vi "Update Graphs.vi"(0 "Select Graph":T15, 2 "appended array":refnum<vi>[](array[refnum]), 5 "ERD Graph  Ind 2":T14, 7 "ERD_Data_Bundled_In":T1, 11 "Error In":errorcluster) -> (1 "All Loads":u16[][](graph), 3 "Water Temperature":dbl(graph), 4 "Basket Speed":u16[][](graph), 6 "Tub Gallons":dbl(graph), 8 "Pressure":dbl(graph), 10 "Motor Current":dbl(graph), 12 "ERD 3":dbl(graph), 13 "ERD 2":dbl(graph), 14 "ERD 1":dbl(graph), 15 "Error Out":errorcluster)   [LabVIEW 2021]
doc: "This VI displays (makes visable) the corresponding graph based on user selection, as well as updates the values of the graphs with current data."
uses:
  type defs/Select _Graph.ctl
  type defs/All_Bundled_Data.ctl
  type defs/Version.ctl
  type defs/ERD_Always_Show.ctl
  type defs/Brass Matrix.ctl
  type defs/CSV_File_String_Arrays.ctl
  type defs/Redundant.ctl
  type defs/Algorithms.ctl
  type defs/ATC_Data.ctl
  type defs/Fault Table Array.ctl
  type defs/Fault_Table_Info.ctl
  Dryer Tool (Commercial 2)/JL Dryer Tool Support/type defs/ERD_RJ45.ctl
  Dryer Tool (Commercial 2)/JL Dryer Tool Support/type defs/ERD_Commercial_Laundry.ctl
  type defs/BootloaderVersion.ctl
panel:
  # "Wet Load Size"
  # "Dry Load Size"
  # "OOB"
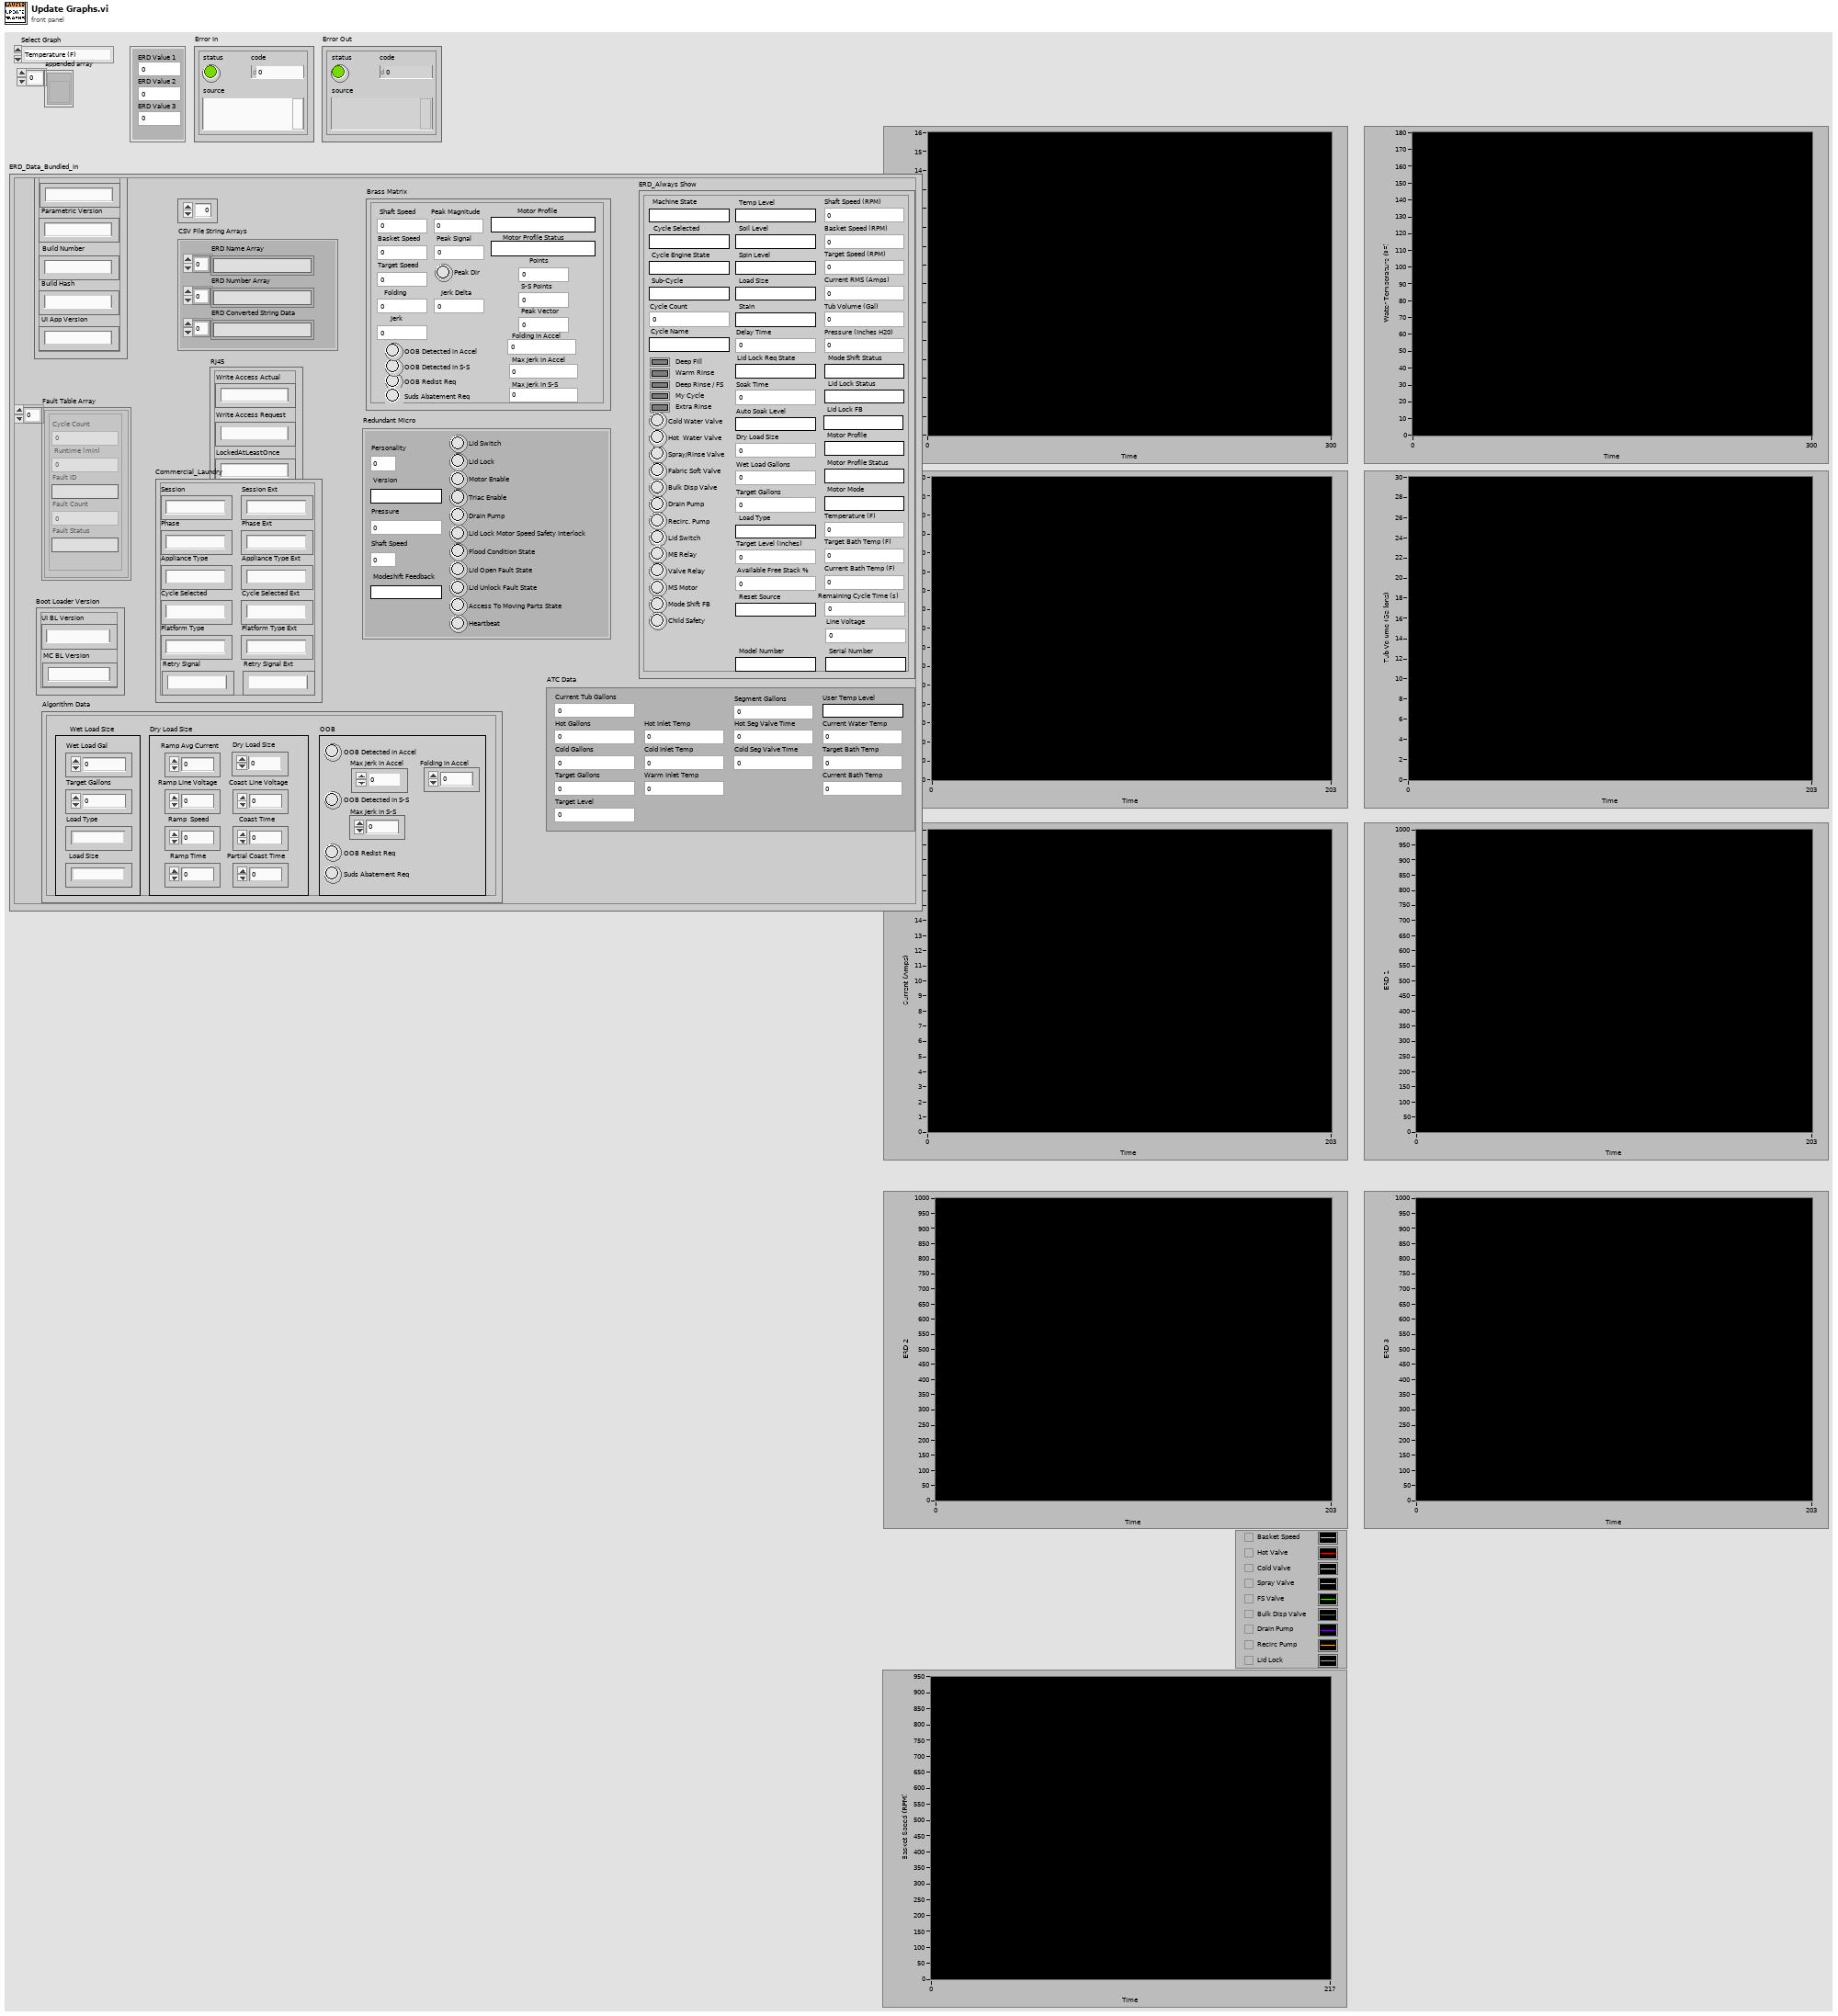
[diagram p1: front panel]
types:
  T1 = typedef "All_Bundled_Data.ctl" = cluster{"Software MC":T2, "ERD_Always Show":T3, "Personality Set":u8, "Brass Matrix":T4, "CSV File String Arrays":T5, "Redundant Micro":T6, "Algorithm Data":T7, "ATC Data":T8, "Fault Table Array ":T9, "RJ45":T11, "Commercial_Laundry":T12, "Boot Loader Version":T13}
  T2 = typedef "Version.ctl" = cluster{"Build Number":string, "Build Hash ":string, "Application Version":string, "Parametric Version":string, "UI App Version":string}
  T3 = typedef "ERD_Always_Show.ctl" = cluster{"Basket Speed (RPM)":u16, "Machine State":string, "Tub Volume (Gal)":dbl, "Pressure (inches H20)":dbl, "Lid Switch ":bool, "Current RMS (Amps)":dbl, "Cycle Selected":string, "Lid Lock Status":string, "Mode Shift Status":string, "Spray/Rinse Valve":bool, "Fabric Soft Valve":bool, "Drain Pump":bool, "Recirc. Pump":bool, "Cycle Engine State":string, "Hot  Water Valve":bool, "Cold Water Valve":bool, "Motor Profile":string, "Motor Profile Status":string, "Motor Mode":string, "ME Relay":bool, "Cycle Count":u32, "Deep Rinse / FS":bool, "My Cycle":bool, "Soil Level":string, "Spin Level":string, "Stain":string, "Temp Level":string, "Load Size":string, "Delay Time":u16, "Soak Time":u16, "Deep Fill":bool, "Warm Rinse":bool, "Auto Soak Level":string, "Extra Rinse":bool, "Wet Load Gallons":dbl, "Target Gallons":dbl, "Sub-Cycle":string, "Load Type":string, "Target Level (inches)":dbl, "Valve Relay":bool, "Dry Load Size":dbl, "Shaft Speed (RPM) ":u16, "MS Motor":bool, "Mode Shift FB":bool, "Target Bath Temp (F)":dbl, "Temperature (F)":dbl, "Current Bath Temp (F)":dbl, "Lid Lock FB":string, "Lid Lock Req State":string, "Remaining Cycle Time (s)":u32, "Available Free Stack %":u8, "Child Safety":bool, "Target Speed (RPM)":u16, "Reset Source":string, "Line Voltage":dbl, "Cycle Name":string, "Bulk Disp Valve":bool, "Model Number":string, "Serial Number":string}
  T4 = typedef "Brass Matrix.ctl" = cluster{"Shaft Speed":u16, "Folding":i32, "Jerk":i32, "Basket Speed":u16, "Target Speed":u16, "Peak Signal":u8, " Peak Magnitude":dbl, "Folding in Accel":i32, "Max Jerk in Accel":i32, "Max Jerk in S-S":i32, "Motor Profile Status":string, "Motor Profile":string, "OOB Redist Req":bool, "OOB Detected in S-S":bool, "OOB Detected in Accel":bool, "Suds Abatement Req ":bool, "Peak Dir":bool, "Peak Vector":dbl, "S-S Points":u8, "Points":u8, "Jerk Delta":i32}
  T5 = typedef "CSV_File_String_Arrays.ctl" = cluster{"ERD Number Array":string[], "ERD Name Array":string[], "ERD Converted String Data":string[]}
  T6 = typedef "Redundant.ctl" = cluster{"Version":string, "Personality":u8, "Pressure ":dbl, "Shaft Speed":u16, "Modeshift Feedback":string, "Lid Switch":bool, "Lid Lock":bool, "Triac Enable":bool, "Drain Pump":bool, "Lid Lock Motor Speed Safety Interlock":bool, "Flood Condition State":bool, "Lid Open Fault State":bool, "Access To Moving Parts State":bool, "Heartbeat":bool, "Motor Enable":bool, "Lid Unlock Fault State":bool}
  T7 = typedef "Algorithms.ctl" = cluster{"Wet Load Gal":dbl, "Target Gallons":dbl, "Load Type":string, "Load Size":string, "Coast Time":u16, "Ramp Time":u16, "Ramp  Speed":u16, "Ramp Avg Current":dbl, "OOB Redist Req":bool, "OOB Detected in S-S":bool, "Folding in Accel":i32, "Max Jerk in Accel":i32, "Max Jerk in S-S":i32, "OOB Detected in Accel":bool, "Partial Coast Time":u16, "Dry Load Size":dbl, "Ramp Line Voltage ":dbl, "Coast Line Voltage":dbl, "Suds Abatement Req ":bool}
  T8 = typedef "ATC_Data.ctl" = cluster{"Current Tub Gallons":dbl, "Hot Gallons":dbl, "Cold Gallons":dbl, "Target Gallons":dbl, "Current Water Temp":dbl, "Target Level":dbl, "Target Bath Temp":dbl, "Current Bath Temp ":dbl, "Cold Inlet Temp":dbl, "Hot Inlet Temp":dbl, "Warm Inlet Temp":dbl, "Hot Seg Valve Time":u16, "Cold Seg Valve Time ":u16, "User Temp Level":string, "Segment Gallons":dbl}
  T9 = typedef "Fault Table Array.ctl" = T10[]
  T10 = typedef "Fault_Table_Info.ctl" = cluster{"Cycle Count":u32, " Runtime (min) ":u32, "Fault Status":string, "Fault ID":string, "Fault Count":u16}
  T11 = typedef "ERD_RJ45.ctl" = cluster{"Write Access Actual":string, "Write Access Request":string, "LockedAtLeastOnce":string}
  T12 = typedef "ERD_Commercial_Laundry.ctl" = cluster{"Session":string, "Phase":string, "Appliance Type":string, "Cycle Selected":string, "Platform Type":string, "Retry Signal":string, "Session Ext":string, "Phase Ext":string, "Appliance Type Ext":string, "Cycle Selected Ext":string, "Platform Type Ext":string, "Retry Signal Ext":string}
  T13 = typedef "BootloaderVersion.ctl" = cluster{"UI BL Version":string, "MC BL Version":string}
  T14 = cluster{"ERD Value 1":dbl, "ERD Value 2":dbl, "ERD Value 3":dbl}
  T15 = typedef "Select _Graph.ctl" = enum16{"Temperature (F)", "Basket Speed (RPM)", "Tub Volume (Gal)", "Pressure (in H2O)", "Current RMS (Amps)", "ERD 1", "ERD 2", "ERD 3", "All Loads"}
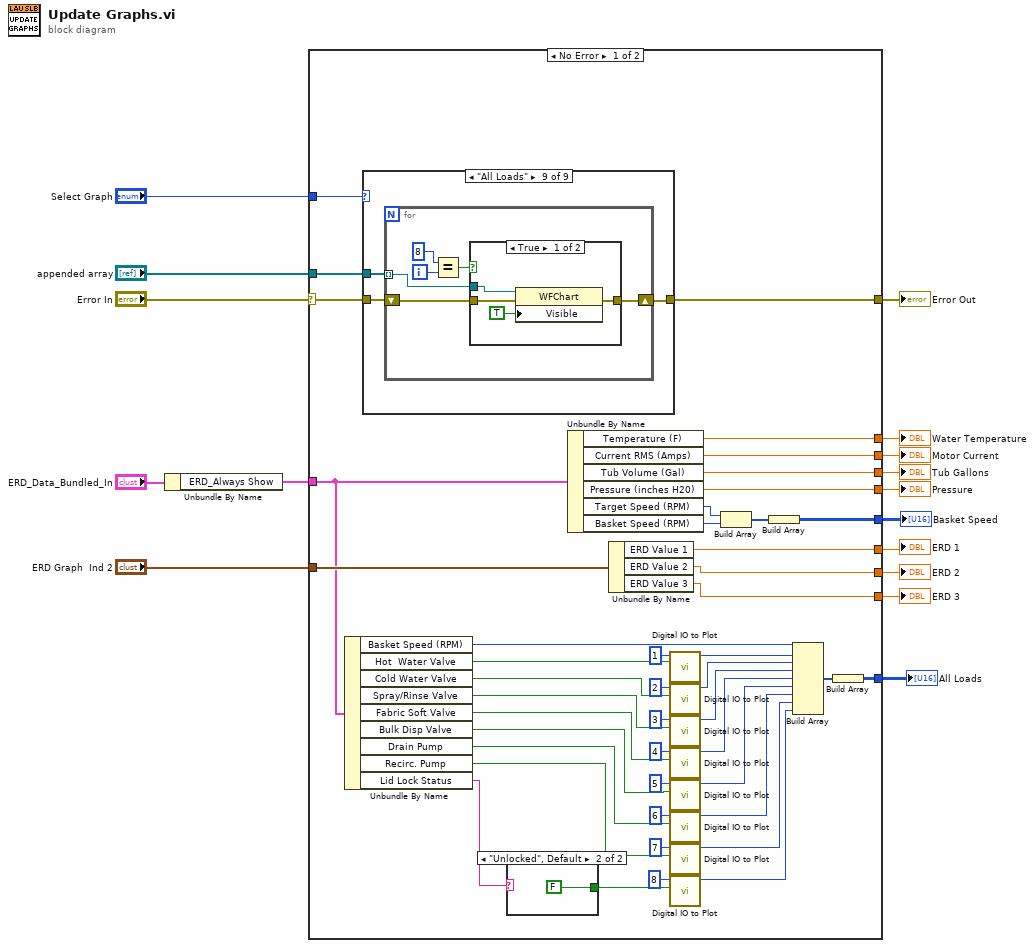
[diagram p0: block diagram]
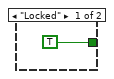
[diagram p2: hidden frame]
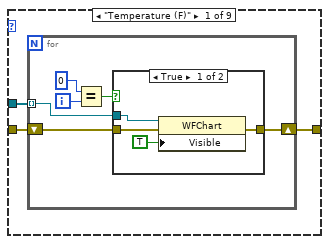
[diagram p3: hidden frame]
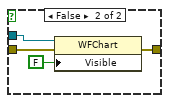
[diagram p4: hidden frame]
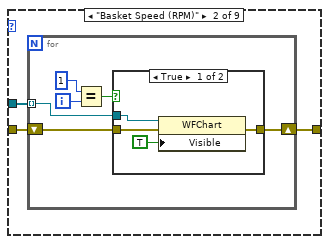
[diagram p5: hidden frame]
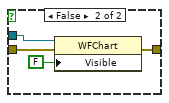
[diagram p6: hidden frame]
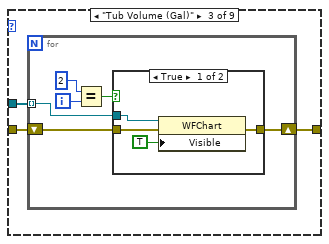
[diagram p7: hidden frame]
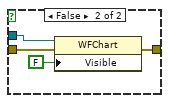
[diagram p8: hidden frame]
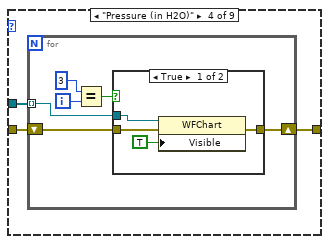
[diagram p9: hidden frame]
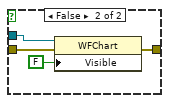
[diagram p10: hidden frame]
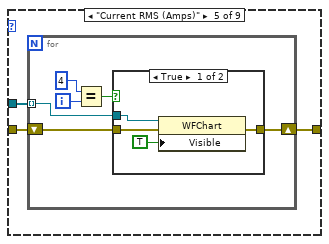
[diagram p11: hidden frame]
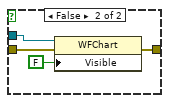
[diagram p12: hidden frame]
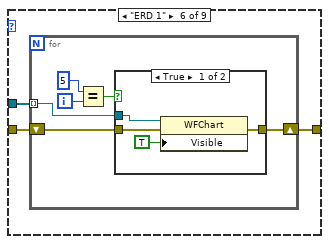
[diagram p13: hidden frame]
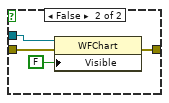
[diagram p14: hidden frame]
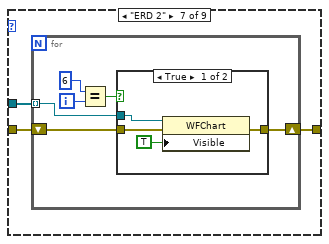
[diagram p15: hidden frame]
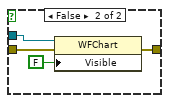
[diagram p16: hidden frame]
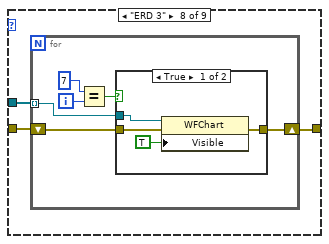
[diagram p17: hidden frame]
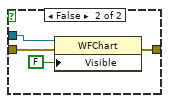
[diagram p18: hidden frame]
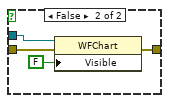
[diagram p19: hidden frame]
diagram:
  n1 = Unbundle By Name("ERD_Data_Bundled_In") -> ("ERD_Always Show"=w3:T3)
  n2 = case shown="No Error" "Error In" {
    selector: "Error In" -> [w59 w217]
    tunnel: [w58 w217] -> w15
    tunnel: w3 -> [w45 _]
    tunnel: "appended array" -> [w60 _]
    tunnel: "Select Graph" -> [w61 _]
    tunnel: [w57 _] -> w12
    tunnel: [w56 _] -> w11
    tunnel: [w55 _] -> w10
    tunnel: [w54 _] -> w9
    tunnel: "ERD Graph  Ind 2" -> [w53 _]
    tunnel: [w52 _] -> w7
    tunnel: [w51 _] -> w6
    tunnel: [w50 _] -> w5
    tunnel: [w46 _] -> w4
    tunnel: [w20 _] -> w1
    frame No Error {
      n3 = Unbundle By Name(w45) -> ("Basket Speed (RPM)"=w44:u16, "Hot  Water Valve"=w43:bool, "Cold Water Valve"=w41:bool, "Spray/Rinse Valve"=w39:bool, "Fabric Soft Valve"=w37:bool, "Bulk Disp Valve"=w17:bool, "Drain Pump"=w35:bool, "Recirc. Pump"=w33:bool, "Lid Lock Status"=w31:string)
      n4 = case shown="\"All Loads\"" w61 {
        tunnel: w60 -> [w66 w83 w100 w117 w133 w150 w168 w183 w200]
        tunnel: w59 -> [w65 w82 w99 w116 w134 w151 w167 w185 w202]
        tunnel: [w64 w81 w98 w115 w132 w149 w166 w184 w201] -> w58
        frame "Temperature (F)" {
          n5 = for {
            tunnel: w66 -> [w72] mode=indexing
            shift-right: [w70] -> w64
            shift-left: w65 -> [w71]
            i -> [w69]
            n6 = Equal?(x=0 ("index"), y=w69) -> (x = y?=w67:bool)
            n7 = case shown="True" w67 {
              tunnel: w72 -> [w76 w80]
              tunnel: w71 -> [w74 w78]
              tunnel: [w73 w77] -> w70
              frame True {
                n8 = property class="WFChart"(reference=w76, error in=w74, "Visible"=TRUE) -> (error out=w73:errorcluster)  [unwired: 1 out]
              }
              frame False {
                n9 = property class="WFChart"(reference=w80, error in=w78, "Visible"=FALSE) -> (error out=w77:errorcluster)  [unwired: 1 out]
              }
            }
          }
        }
        frame "Basket Speed (RPM)" {
          n10 = for {
            tunnel: w83 -> [w89] mode=indexing
            shift-right: [w87] -> w81
            shift-left: w82 -> [w88]
            i -> [w86]
            n11 = Equal?(x=1 ("index"), y=w86) -> (x = y?=w84:bool)
            n12 = case shown="True" w84 {
              tunnel: w89 -> [w93 w97]
              tunnel: w88 -> [w91 w95]
              tunnel: [w90 w94] -> w87
              frame True {
                n13 = property class="WFChart"(reference=w93, error in=w91, "Visible"=TRUE) -> (error out=w90:errorcluster)  [unwired: 1 out]
              }
              frame False {
                n14 = property class="WFChart"(reference=w97, error in=w95, "Visible"=FALSE) -> (error out=w94:errorcluster)  [unwired: 1 out]
              }
            }
          }
        }
        frame "Tub Volume (Gal)" {
          n15 = for {
            tunnel: w100 -> [w106] mode=indexing
            shift-right: [w104] -> w98
            shift-left: w99 -> [w105]
            i -> [w103]
            n16 = Equal?(x=2 ("index"), y=w103) -> (x = y?=w101:bool)
            n17 = case shown="True" w101 {
              tunnel: w106 -> [w110 w114]
              tunnel: w105 -> [w108 w112]
              tunnel: [w107 w111] -> w104
              frame True {
                n18 = property class="WFChart"(reference=w110, error in=w108, "Visible"=TRUE) -> (error out=w107:errorcluster)  [unwired: 1 out]
              }
              frame False {
                n19 = property class="WFChart"(reference=w114, error in=w112, "Visible"=FALSE) -> (error out=w111:errorcluster)  [unwired: 1 out]
              }
            }
          }
        }
        frame "Pressure (in H2O)" {
          n20 = for {
            tunnel: w117 -> [w123] mode=indexing
            shift-right: [w121] -> w115
            shift-left: w116 -> [w122]
            i -> [w120]
            n21 = Equal?(x=3 ("index"), y=w120) -> (x = y?=w118:bool)
            n22 = case shown="True" w118 {
              tunnel: w123 -> [w127 w131]
              tunnel: w122 -> [w125 w129]
              tunnel: [w124 w128] -> w121
              frame True {
                n23 = property class="WFChart"(reference=w127, error in=w125, "Visible"=TRUE) -> (error out=w124:errorcluster)  [unwired: 1 out]
              }
              frame False {
                n24 = property class="WFChart"(reference=w131, error in=w129, "Visible"=FALSE) -> (error out=w128:errorcluster)  [unwired: 1 out]
              }
            }
          }
        }
        frame "Current RMS (Amps)" {
          n25 = for {
            tunnel: w133 -> [w140] mode=indexing
            shift-right: [w138] -> w132
            shift-left: w134 -> [w139]
            i -> [w137]
            n26 = Equal?(x=4 ("index"), y=w137) -> (x = y?=w135:bool)
            n27 = case shown="True" w135 {
              tunnel: w140 -> [w144 w148]
              tunnel: w139 -> [w142 w146]
              tunnel: [w141 w145] -> w138
              frame True {
                n28 = property class="WFChart"(reference=w144, error in=w142, "Visible"=TRUE) -> (error out=w141:errorcluster)  [unwired: 1 out]
              }
              frame False {
                n29 = property class="WFChart"(reference=w148, error in=w146, "Visible"=FALSE) -> (error out=w145:errorcluster)  [unwired: 1 out]
              }
            }
          }
        }
        frame "ERD 1" {
          n30 = for {
            tunnel: w150 -> [w157] mode=indexing
            shift-right: [w155] -> w149
            shift-left: w151 -> [w156]
            i -> [w154]
            n31 = Equal?(x=5 ("index"), y=w154) -> (x = y?=w152:bool)
            n32 = case shown="True" w152 {
              tunnel: w157 -> [w161 w165]
              tunnel: w156 -> [w159 w163]
              tunnel: [w158 w162] -> w155
              frame True {
                n33 = property class="WFChart"(reference=w161, error in=w159, "Visible"=TRUE) -> (error out=w158:errorcluster)  [unwired: 1 out]
              }
              frame False {
                n34 = property class="WFChart"(reference=w165, error in=w163, "Visible"=FALSE) -> (error out=w162:errorcluster)  [unwired: 1 out]
              }
            }
          }
        }
        frame "ERD 2" {
          n35 = for {
            tunnel: w168 -> [w174] mode=indexing
            shift-right: [w172] -> w166
            shift-left: w167 -> [w173]
            i -> [w171]
            n36 = Equal?(x=6 ("index"), y=w171) -> (x = y?=w169:bool)
            n37 = case shown="True" w169 {
              tunnel: w174 -> [w178 w182]
              tunnel: w173 -> [w176 w180]
              tunnel: [w175 w179] -> w172
              frame True {
                n38 = property class="WFChart"(reference=w178, error in=w176, "Visible"=TRUE) -> (error out=w175:errorcluster)  [unwired: 1 out]
              }
              frame False {
                n39 = property class="WFChart"(reference=w182, error in=w180, "Visible"=FALSE) -> (error out=w179:errorcluster)  [unwired: 1 out]
              }
            }
          }
        }
        frame "ERD 3" {
          n40 = for {
            tunnel: w183 -> [w191] mode=indexing
            shift-right: [w189] -> w184
            shift-left: w185 -> [w190]
            i -> [w188]
            n41 = Equal?(x=7 ("index"), y=w188) -> (x = y?=w186:bool)
            n42 = case shown="True" w186 {
              tunnel: w191 -> [w195 w199]
              tunnel: w190 -> [w193 w197]
              tunnel: [w192 w196] -> w189
              frame True {
                n43 = property class="WFChart"(reference=w195, error in=w193, "Visible"=TRUE) -> (error out=w192:errorcluster)  [unwired: 1 out]
              }
              frame False {
                n44 = property class="WFChart"(reference=w199, error in=w197, "Visible"=FALSE) -> (error out=w196:errorcluster)  [unwired: 1 out]
              }
            }
          }
        }
        frame "All Loads" {
          n45 = for {
            tunnel: w200 -> [w208] mode=indexing
            shift-right: [w206] -> w201
            shift-left: w202 -> [w207]
            i -> [w205]
            n46 = Equal?(x=8 ("index"), y=w205) -> (x = y?=w203:bool)
            n47 = case shown="True" w203 {
              tunnel: w208 -> [w212 w216]
              tunnel: w207 -> [w210 w214]
              tunnel: [w209 w213] -> w206
              frame True {
                n48 = property class="WFChart"(reference=w212, error in=w210, "Visible"=TRUE) -> (error out=w209:errorcluster)  [unwired: 1 out]
              }
              frame False {
                n49 = property class="WFChart"(reference=w216, error in=w214, "Visible"=FALSE) -> (error out=w213:errorcluster)  [unwired: 1 out]
              }
            }
          }
        }
      }
      n50 = case shown="\"Unlocked\", Default" w31 {
        tunnel: [TRUE FALSE] -> w29
        frame "Locked" {
        }
        frame "Unlocked", Default {
        }
      }
      n51 = Unbundle By Name(w45) -> ("Temperature (F)"=w57:dbl, "Current RMS (Amps)"=w56:dbl, "Tub Volume (Gal)"=w55:dbl, "Pressure (inches H20)"=w54:dbl, "Target Speed (RPM)"=w49:u16, "Basket Speed (RPM)"=w48:u16)
      n52 = Unbundle By Name(w53) -> ("ERD Value 1"=w52:dbl, "ERD Value 2"=w51:dbl, "ERD Value 3"=w50:dbl)
      n53 = call "Digital IO to Plot.vi"("Boolean Value"=w43, "Multiplier"=u16 1) -> ("Output"=w28:u16)  [unwired: 9 in]
      n54 = call "Digital IO to Plot.vi"("Boolean Value"=w41, "Multiplier"=u16 2) -> ("Output"=w27:u16)  [unwired: 9 in]
      n55 = call "Digital IO to Plot.vi"("Boolean Value"=w39, "Multiplier"=u16 3) -> ("Output"=w26:u16)  [unwired: 9 in]
      n56 = call "Digital IO to Plot.vi"("Boolean Value"=w37, "Multiplier"=u16 4) -> ("Output"=w25:u16)  [unwired: 9 in]
      n57 = call "Digital IO to Plot.vi"("Boolean Value"=w17, "Multiplier"=u16 5) -> ("Output"=w18:u16)  [unwired: 9 in]
      n58 = call "Digital IO to Plot.vi"("Boolean Value"=w35, "Multiplier"=u16 6) -> ("Output"=w24:u16)  [unwired: 9 in]
      n59 = call "Digital IO to Plot.vi"("Boolean Value"=w33, "Multiplier"=u16 7) -> ("Output"=w23:u16)  [unwired: 9 in]
      n60 = call "Digital IO to Plot.vi"("Boolean Value"=w29, "Multiplier"=u16 8) -> ("Output"=w22:u16)  [unwired: 9 in]
      n61 = Build Array(w49, w48) -> (w47:u16[])
      n62 = Build Array(w47) -> (w46:u16[][])
      n63 = Build Array(w44, w28, w27, w26, w25, w18, w24, w23, w22) -> (w21:u16[])
      n64 = Build Array(w21) -> (w20:u16[][])
    }
    frame Error {
    }
  }
  "Error Out" <- w15
  "Water Temperature" <- w12
  "Basket Speed" <- w4
  "Motor Current" <- w11
  "Tub Gallons" <- w10
  "Pressure" <- w9
  "ERD 1" <- w7
  "ERD 2" <- w6
  "ERD 3" <- w5
  "All Loads" <- w1
